vi "sendWaitForAnswer.vi"(8 "error in (no error)":errorcluster, 10 "message":string, 11 "NetworkServer in":refnum<class "NetworkServer.lvclass">) -> (0 "error out":errorcluster, 1 "valid?":bool[](array[boolean]), 2 "answers":string[](array[string]), 3 "NetworkServer out":refnum<class "NetworkServer.lvclass">)   [LabVIEW 2011, in "Hardware.lvlib" / "HWControllers.lvlib" / "NetworkServer.lvclass"]
uses:
  NetworkServer.lvclass
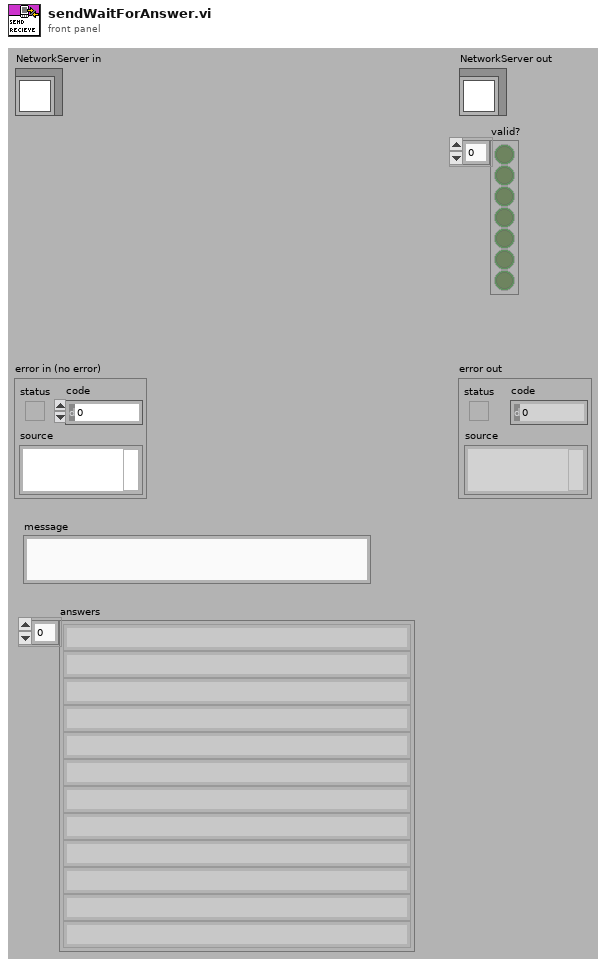
[diagram p1: front panel]
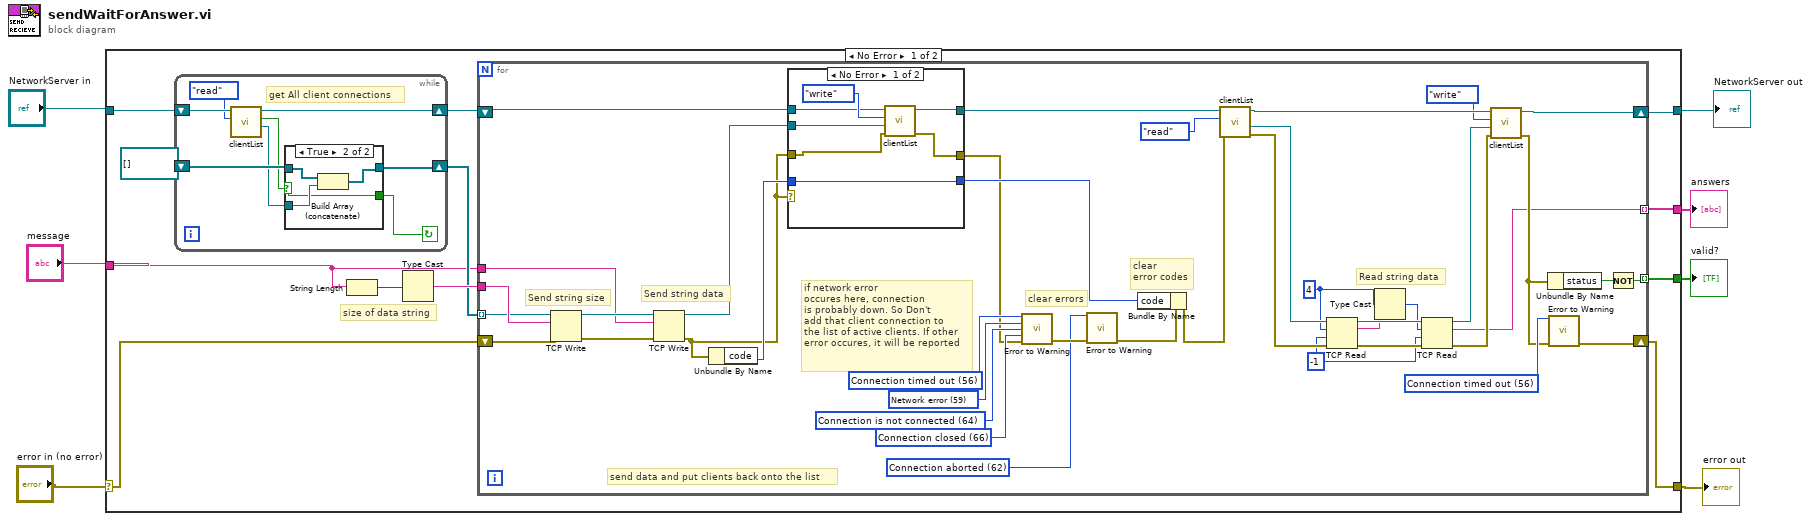
[diagram p0: block diagram]
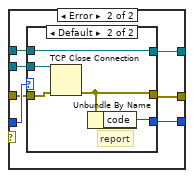
[diagram p2: hidden frame]
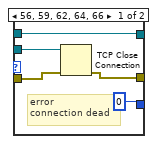
[diagram p3: hidden frame]
diagram:
  n1 = case shown="No Error" "error in (no error)" {
    selector: "error in (no error)" -> [w13 w100]
    tunnel: [w15 w100] -> w1
    tunnel: [w10 w99] -> w4
    tunnel: "NetworkServer in" -> [w12 w99]
    tunnel: "message" -> [w14 _]
    tunnel: [w9 _] -> w2
    tunnel: [w8 _] -> w3
    frame No Error {
      # "size of data string"
      n2 = while {
        shift-right: [w90] -> w16
        shift-left: refnum<k5>[] [] ("empty") -> [w91]
        shift-right: [w86] -> w11
        shift-left: w12 -> [w89]
        stop <- w92 continue-if-true
        # "get All client connections"
        n3 = call "clientList.vi"("Enum"=enum16{"read", "write", "reset"}."read", "NetworkServer in"=w89) -> ("client"=w87:refnum<k5>, "valid?"=w88:bool, "NetworkServer out"=w86:refnum<class "NetworkServer.lvclass">)  [unwired: 6 in, 1 out]
        n4 = case shown="True" w88 {
          selector: w88 -> [w93 w96]
          tunnel: w87 -> [_ w98]
          tunnel: w91 -> [w94 w97]
          tunnel: [w93 w96] -> w92
          tunnel: [w94 w95] -> w90
          frame False {
          }
          frame True {
            n5 = Build Array (concatenate)(w97, w98) -> (w95:refnum<k5>[])
          }
        }
      }
      n6 = String Length(string=w14) -> (length=w18:i32)
      n7 = Type Cast(x=w18) -> (*(type *) &x=w19:string)  [unwired: 1 in]
      n8 = for {
        tunnel: w19 -> [w58]
        tunnel: w14 -> [w57]
        tunnel: w16 -> [w55] mode=indexing
        shift-right: [w32] -> w15
        shift-left: w13 -> [w56]
        shift-right: [w37] -> w10
        shift-left: w11 -> [w54]
        tunnel: [w28] -> w9 mode=indexing
        tunnel: [w29] -> w8 mode=indexing
        w20 = -1
        w33 = 56 items=["No Error", "Argument Error", "Memory Full", "Out of Zone", "End of File", "File Already Open", "Generic File IO Error", "File Not Found", "File Permission Error", "Disk Full", "Duplicate Path", "Too Many Files Open", "Not Enabled", "Resource File Not Found", "Cannot Add Resource", "Resource Not Found", "Image Not Found", "Image Memory Error", "Pen Does Not Exist", "Config Bad Type", "Config Token Not Found", "Config Parse Error", "Config Memory Error", "Bad External Code Format", "Bad External Code Offset", "External Code Not Present", "Null Window", "Destroy Window Mixup", "Null Menu", "Print Aborted", "Bad Print Record", "Print Driver Error", "Windows Error During Print", "Memory Error During Print", "Print Dialog Error", "Generic Print Error", "Invalid Device Refnum", "Device Not Found", "Device Parameter Error", "Device Unit Error", "Can't Open Device", "Device Call Aborted", "Generic Error", "Cancelled By User", "Object ID Too Low", "Object ID Too High", "Object Not In Heap", "Unknown Heap", "Bad DefProc ID", "DefProc Not In Table", "Message Out Of Range", "Null Method", "Unknown Message", "Manager Call Not Supported", "Bad address", "Connection In progress", "Connection timed out", "Connection is already in progress", "Network attribute not supported", "Network error", "Address in use", "System out of memory", "Connection aborted", "Connection refused", "Connection is not connected", "Connection is already connected", "Connection closed", "Initialize error (interapplication manager)", "Bad occurrence", "Wait on unbound occurrence handler", "Occurrence queue overflow", "Bad path", "Semaphore not signaled", "Unrecognized type (interapplication manager)"] ("1st Error to Convert")
        w24 = 4
        w46 = 62 items=["No Error", "Argument Error", "Memory Full", "Out of Zone", "End of File", "File Already Open", "Generic File IO Error", "File Not Found", "File Permission Error", "Disk Full", "Duplicate Path", "Too Many Files Open", "Not Enabled", "Resource File Not Found", "Cannot Add Resource", "Resource Not Found", "Image Not Found", "Image Memory Error", "Pen Does Not Exist", "Config Bad Type", "Config Token Not Found", "Config Parse Error", "Config Memory Error", "Bad External Code Format", "Bad External Code Offset", "External Code Not Present", "Null Window", "Destroy Window Mixup", "Null Menu", "Print Aborted", "Bad Print Record", "Print Driver Error", "Windows Error During Print", "Memory Error During Print", "Print Dialog Error", "Generic Print Error", "Invalid Device Refnum", "Device Not Found", "Device Parameter Error", "Device Unit Error", "Can't Open Device", "Device Call Aborted", "Generic Error", "Cancelled By User", "Object ID Too Low", "Object ID Too High", "Object Not In Heap", "Unknown Heap", "Bad DefProc ID", "DefProc Not In Table", "Message Out Of Range", "Null Method", "Unknown Message", "Manager Call Not Supported", "Bad address", "Connection In progress", "Connection timed out", "Connection is already in progress", "Network attribute not supported", "Network error", "Address in use", "System out of memory", "Connection aborted", "Connection refused", "Connection is not connected", "Connection is already connected", "Connection closed", "Initialize error (interapplication manager)", "Bad occurrence", "Wait on unbound occurrence handler", "Occurrence queue overflow", "Bad path", "Semaphore not signaled", "Unrecognized type (interapplication manager)"] ("1st Error to Convert")
        w51 = 56 items=["No Error", "Argument Error", "Memory Full", "Out of Zone", "End of File", "File Already Open", "Generic File IO Error", "File Not Found", "File Permission Error", "Disk Full", "Duplicate Path", "Too Many Files Open", "Not Enabled", "Resource File Not Found", "Cannot Add Resource", "Resource Not Found", "Image Not Found", "Image Memory Error", "Pen Does Not Exist", "Config Bad Type", "Config Token Not Found", "Config Parse Error", "Config Memory Error", "Bad External Code Format", "Bad External Code Offset", "External Code Not Present", "Null Window", "Destroy Window Mixup", "Null Menu", "Print Aborted", "Bad Print Record", "Print Driver Error", "Windows Error During Print", "Memory Error During Print", "Print Dialog Error", "Generic Print Error", "Invalid Device Refnum", "Device Not Found", "Device Parameter Error", "Device Unit Error", "Can't Open Device", "Device Call Aborted", "Generic Error", "Cancelled By User", "Object ID Too Low", "Object ID Too High", "Object Not In Heap", "Unknown Heap", "Bad DefProc ID", "DefProc Not In Table", "Message Out Of Range", "Null Method", "Unknown Message", "Manager Call Not Supported", "Bad address", "Connection In progress", "Connection timed out", "Connection is already in progress", "Network attribute not supported", "Network error", "Address in use", "System out of memory", "Connection aborted", "Connection refused", "Connection is not connected", "Connection is already connected", "Connection closed", "Initialize error (interapplication manager)", "Bad occurrence", "Wait on unbound occurrence handler", "Occurrence queue overflow", "Bad path", "Semaphore not signaled", "Unrecognized type (interapplication manager)"] ("1st Error to Convert")
        w50 = 59 items=["No Error", "Argument Error", "Memory Full", "Out of Zone", "End of File", "File Already Open", "Generic File IO Error", "File Not Found", "File Permission Error", "Disk Full", "Duplicate Path", "Too Many Files Open", "Not Enabled", "Resource File Not Found", "Cannot Add Resource", "Resource Not Found", "Image Not Found", "Image Memory Error", "Pen Does Not Exist", "Config Bad Type", "Config Token Not Found", "Config Parse Error", "Config Memory Error", "Bad External Code Format", "Bad External Code Offset", "External Code Not Present", "Null Window", "Destroy Window Mixup", "Null Menu", "Print Aborted", "Bad Print Record", "Print Driver Error", "Windows Error During Print", "Memory Error During Print", "Print Dialog Error", "Generic Print Error", "Invalid Device Refnum", "Device Not Found", "Device Parameter Error", "Device Unit Error", "Can't Open Device", "Device Call Aborted", "Generic Error", "Cancelled By User", "Object ID Too Low", "Object ID Too High", "Object Not In Heap", "Unknown Heap", "Bad DefProc ID", "DefProc Not In Table", "Message Out Of Range", "Null Method", "Unknown Message", "Manager Call Not Supported", "Bad address", "Connection In progress", "Connection timed out", "Connection is already in progress", "Network attribute not supported", "Network error", "Address in use", "System out of memory", "Connection aborted", "Connection refused", "Connection is not connected", "Connection is already connected", "Connection closed", "Initialize error (interapplication manager)", "Bad occurrence", "Wait on unbound occurrence handler", "Occurrence queue overflow", "Bad path", "Semaphore not signaled", "Unrecognized type (interapplication manager)"] ("1st Error to Convert")
        w48 = 66 items=["No Error", "Argument Error", "Memory Full", "Out of Zone", "End of File", "File Already Open", "Generic File IO Error", "File Not Found", "File Permission Error", "Disk Full", "Duplicate Path", "Too Many Files Open", "Not Enabled", "Resource File Not Found", "Cannot Add Resource", "Resource Not Found", "Image Not Found", "Image Memory Error", "Pen Does Not Exist", "Config Bad Type", "Config Token Not Found", "Config Parse Error", "Config Memory Error", "Bad External Code Format", "Bad External Code Offset", "External Code Not Present", "Null Window", "Destroy Window Mixup", "Null Menu", "Print Aborted", "Bad Print Record", "Print Driver Error", "Windows Error During Print", "Memory Error During Print", "Print Dialog Error", "Generic Print Error", "Invalid Device Refnum", "Device Not Found", "Device Parameter Error", "Device Unit Error", "Can't Open Device", "Device Call Aborted", "Generic Error", "Cancelled By User", "Object ID Too Low", "Object ID Too High", "Object Not In Heap", "Unknown Heap", "Bad DefProc ID", "DefProc Not In Table", "Message Out Of Range", "Null Method", "Unknown Message", "Manager Call Not Supported", "Bad address", "Connection In progress", "Connection timed out", "Connection is already in progress", "Network attribute not supported", "Network error", "Address in use", "System out of memory", "Connection aborted", "Connection refused", "Connection is not connected", "Connection is already connected", "Connection closed", "Initialize error (interapplication manager)", "Bad occurrence", "Wait on unbound occurrence handler", "Occurrence queue overflow", "Bad path", "Semaphore not signaled", "Unrecognized type (interapplication manager)"] ("2nd Error to Convert")
        w49 = 64 items=["No Error", "Argument Error", "Memory Full", "Out of Zone", "End of File", "File Already Open", "Generic File IO Error", "File Not Found", "File Permission Error", "Disk Full", "Duplicate Path", "Too Many Files Open", "Not Enabled", "Resource File Not Found", "Cannot Add Resource", "Resource Not Found", "Image Not Found", "Image Memory Error", "Pen Does Not Exist", "Config Bad Type", "Config Token Not Found", "Config Parse Error", "Config Memory Error", "Bad External Code Format", "Bad External Code Offset", "External Code Not Present", "Null Window", "Destroy Window Mixup", "Null Menu", "Print Aborted", "Bad Print Record", "Print Driver Error", "Windows Error During Print", "Memory Error During Print", "Print Dialog Error", "Generic Print Error", "Invalid Device Refnum", "Device Not Found", "Device Parameter Error", "Device Unit Error", "Can't Open Device", "Device Call Aborted", "Generic Error", "Cancelled By User", "Object ID Too Low", "Object ID Too High", "Object Not In Heap", "Unknown Heap", "Bad DefProc ID", "DefProc Not In Table", "Message Out Of Range", "Null Method", "Unknown Message", "Manager Call Not Supported", "Bad address", "Connection In progress", "Connection timed out", "Connection is already in progress", "Network attribute not supported", "Network error", "Address in use", "System out of memory", "Connection aborted", "Connection refused", "Connection is not connected", "Connection is already connected", "Connection closed", "Initialize error (interapplication manager)", "Bad occurrence", "Wait on unbound occurrence handler", "Occurrence queue overflow", "Bad path", "Semaphore not signaled", "Unrecognized type (interapplication manager)"] ("1st Error to Convert")
        # "Read string data"
        # "clear\nerror codes"
        # "clear errors"
        # "if network error \noccures here, connection\nis probably down. So Don't\nadd that client connection to\nthe list of active clients. If other\nerror occures, it will be reported"
        # "send data and put clients back onto the list"
        # "Send string data"
        # "Send string size"
        n9 = TCP Write(connection ID=w55, data in=w58, error in (no error)=w56) -> (connection ID out=w59:refnum<k5>, error out=w60:errorcluster)  [unwired: 1 in, 1 out]
        n10 = TCP Write(connection ID=w59, data in=w57, error in (no error)=w60) -> (connection ID out=w53:refnum<k5>, error out=w22:errorcluster)  [unwired: 1 in, 1 out]
        n11 = Unbundle By Name(w22) -> ("code"=w52:i32)
        n12 = case shown="No Error" w22 {
          tunnel: w54 -> [w66 w74]
          tunnel: w53 -> [w62 w73]
          tunnel: w52 -> [w61 w72]
          tunnel: w22 -> [w64 w71]
          tunnel: [w63 w70] -> w21
          tunnel: [w61 w69] -> w44
          tunnel: [w65 w68] -> w43
          frame No Error {
            n13 = call "clientList.vi"("error in (no error)"=w64, "new client"=w62, "Enum"=enum16{"read", "write", "reset"}."write", "NetworkServer in"=w66) -> ("error out"=w63:errorcluster, "NetworkServer out"=w65:refnum<class "NetworkServer.lvclass">)  [unwired: 4 in, 2 out]
          }
          frame Error {
            n14 = case shown="Default" w72 {
              tunnel: [w79 w82] -> w68
              tunnel: w74 -> [w79 w82]
              tunnel: w73 -> [w78 w84]
              tunnel: w71 -> [w77 w83]
              tunnel: [w76 w81] -> w70
              tunnel: [0 w80] -> w69
              frame 56, 59, 62, 64, 66 {
                # "error\nconnection dead"
                n15 = TCP Close Connection(connection ID=w78, error in (no error)=w77) -> (error out=w76:errorcluster)  [unwired: 1 in, 1 out]
              }
              frame Default {
                # "report"
                n16 = TCP Close Connection(connection ID=w84, error in (no error)=w83) -> (error out=w81:errorcluster)  [unwired: 1 in, 1 out]
                n17 = Unbundle By Name(w81) -> ("code"=w80:i32)
              }
            }
          }
        }
        n18 = call <vilib>:"Error to Warning.vi"("1st Error to Convert"=w51, "2nd Error to Convert"=w50, "3rd Error to Convert"=w49, "4th Error to Convert"=w48, "error in"=w21) -> ("warning out"=w47:errorcluster)  [unwired: 10 out]
        n19 = call <vilib>:"Error to Warning.vi"("1st Error to Convert"=w46, "error in"=w47) -> ("warning out"=w45:errorcluster)  [unwired: 3 in, 10 out]
        n20 = Bundle By Name(cluster=w45, "code"=w44) -> (w42:errorcluster)
        n21 = call "clientList.vi"("error in (no error)"=w42, "Enum"=enum16{"read", "write", "reset"}."read", "NetworkServer in"=w43) -> ("error out"=w38:errorcluster, "client"=w39:refnum<k5>, "NetworkServer out"=w36:refnum<class "NetworkServer.lvclass">)  [unwired: 5 in, 1 out]
        n22 = TCP Read(connection ID=w39, bytes to read=w24, error in (no error)=w38, 9:w20) -> (connection ID out=w40:refnum<k5>, data out=w25:string, error out=w41:errorcluster)  [unwired: 1 out]
        n23 = Type Cast(type=w24, x=w25) -> (*(type *) &x=w23:i32)
        n24 = TCP Read(connection ID=w40, bytes to read=w23, error in (no error)=w41, 9:w20) -> (connection ID out=w35:refnum<k5>, data out=w29:string, error out=w34:errorcluster)  [unwired: 1 out]
        n25 = call "clientList.vi"("error in (no error)"=w34, "new client"=w35, "Enum"=enum16{"read", "write", "reset"}."write", "NetworkServer in"=w36) -> ("error out"=w31:errorcluster, "NetworkServer out"=w37:refnum<class "NetworkServer.lvclass">)  [unwired: 4 in, 2 out]
        n26 = Unbundle By Name(w31) -> ("status"=w30:bool)
        n27 = call <vilib>:"Error to Warning.vi"("1st Error to Convert"=w33, "error in"=w31) -> ("warning out"=w32:errorcluster)  [unwired: 3 in, 10 out]
        n28 = Not(x=w30) -> (.not. x?=w28:bool)
      }
    }
    frame Error {
    }
  }
  "error out" <- w1
  "NetworkServer out" <- w4
  "answers" <- w3
  "valid?" <- w2
